vi "ExTestCCDdim1.vi"() -> ()   [LabVIEW 2010]
panel:
  out "Y dimension":u32
  out "Y dimension programed":u32
  out "X dimension":u32
  out "X dimension programed":u32
  out "error out":errorcluster
  in  "error in (no error)":errorcluster
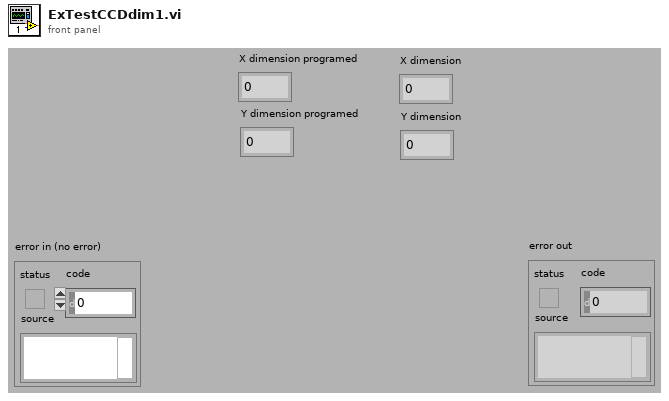
[diagram p1: front panel]
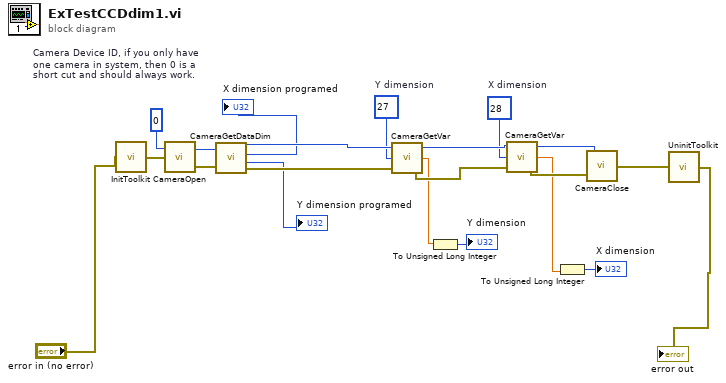
[diagram p0: block diagram]
diagram:
  w7 = 28  # X dimension
  w8 = 27  # Y dimension
  w20 = 0  # Camera Device ID, if you only have  one camera in system, then 0 is a  short cut and should always work.
  n1 = call <userlib>:"InitToolkit.vi"("error in"="error in (no error)") -> ("error out"=w21:errorcluster)
  n2 = call <userlib>:"CameraOpen.vi"("error in"=w21, "Camera Device ID"=w20) -> ("error out"=w16:errorcluster, "Camera Handle"=w15:u32)
  n3 = call <userlib>:"CameraGetDataDim.vi"("Camera Handle"=w15, "error in"=w16) -> ("Camera Handle"=w14:u32, "Xdim"=→"X dimension programed":u32, "Ydim"=→"Y dimension programed":u32, "error out"=w13:errorcluster)
  n4 = call <userlib>:"CameraGetVar.vi"("error in"=w13, "Parameter ID"=w8, "Camera Handle"=w14) -> ("error out"=w12:errorcluster, "Value"=w1:dbl, "Camera Handle"=w10:u32)
  n5 = To Unsigned Long Integer(number=w1) -> (unsigned 32bit integer=→"Y dimension":u32)
  n6 = call <userlib>:"CameraGetVar.vi"("error in"=w12, "Parameter ID"=w7, "Camera Handle"=w10) -> ("error out"=w11:errorcluster, "Value"=w2:dbl, "Camera Handle"=w9:u32)
  n7 = To Unsigned Long Integer(number=w2) -> (unsigned 32bit integer=→"X dimension":u32)
  n8 = call <userlib>:"CameraClose.vi"("error in"=w11, "Camera Handle"=w9) -> ("error out"=w17:errorcluster)
  n9 = call <userlib>:"UninitToolkit.vi"("error in"=w17) -> ("error out"=→"error out":errorcluster)
